vi "WSVCAP SHL FPGA LL Procedure RFFE - Receive Data.vi"(0 "Procedure Step":T1, 1 "Wait Ticks Remaining":u32, 2 "Start of Procedure":bool, 5 "RFFE Wait Ticks":u32, 7 "Read Bits Remaining":u8, 9 "Read Bytes Remaining":u8, 11 "error in (no error)":errorcluster, 12 "RFFE Cycle CMD":u64, 13 "Socket Mask":u64) -> (3 "Wait Ticks Remaining Out":u32, 4 "Procedure Step Out":T1, 6 "Read Bytes Remaining Out":u8, 8 "Read Bits Remaining Out":u8, 10 "Finished":bool, 15 "error out":errorcluster)   [LabVIEW 2017]
uses:
  Type Defs/WSVCAP SHL Procedure Step Enum.ctl
  Type Defs/WSVCAP SHL RFFE Write Line Enum.ctl
  Type Defs/WSVCAP SHL FIFO Operation Enum.ctl
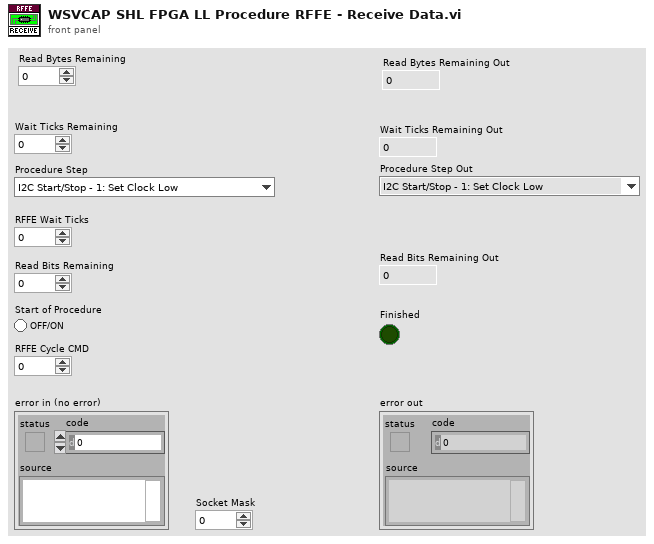
[diagram p1: front panel]
types:
  T1 = typedef "WSVCAP SHL Procedure Step Enum.ctl" = enum16{"I2C Start/Stop - 1: Set Clock Low", "I2C Start/Stop - 2: Wait", "I2C Start/Stop - 3: Set Data I", "I2C Start/Stop - 4: Wait", "I2C Start/Stop - 5: Set Clock High", "I2C Start/Stop - 6: Wait", "I2C Start/Stop - 7: Set Data II", "I2C Start/Stop - 8: Wait", "I2C Start/Stop - 9: Set Clock Low", "I2C Start/Stop - 10: Wait", "I2C Read ACK - 1: Set Clock High", "I2C Read ACK - 2: Wait", "I2C Read ACK - 3: Read ACK Bit", "I2C Read ACK - 4: Wait", "I2C Read ACK - 5: Set Clock Low", "I2C Read ACK - 6: Wait", "I2C Write ACK - 1: Write ACK Bit", "I2C Write ACK - 2: Wait", "I2C Write ACK - 3: Set Clock High", "I2C Write ACK - 4: Wait", "I2C Write ACK - 5: Set Clock Low", "I2C Write ACK - 6: Wait", "I2C Write ACK - 7: Set Data Low", "I2C Send Add - 1: Reset Bits Remaining", "I2C Send Add - 2: Set Data Bit", "I2C Send Add - 3: Wait", "I2C Send Add - 4: Set Clock High", "I2C Send Add - 5: Wait", "I2C Send Add - 6: Set Clock Low", "I2C Send Add - 7: Wait", "I2C Send Add - 8: Check Bits Remaining", "I2C Send Data - 1: Reset Bits Remaining", "I2C Send Data - 2: Load Write Bit from FIFO", "I2C Send Data - 3: Set Data Bit", "I2C Send Data - 4: Wait", "I2C Send Data - 5: Set Clock High", "I2C Send Data - 6: Wait", "I2C Send Data - 7: Set Clock Low", "I2C Send Data - 8: Wait", "I2C Send Data - 9: Check Bits Remaining", "I2C Receive Data - 1: Reset Bits Remaining", "I2C Receive Data - 2: Wait", "I2C Receive Data - 3: Set Clock High", "I2C Receive Data - 4: Wait", "I2C Receive Data - 5: Read Data Bit", "I2C Receive Data - 6: Wait", "I2C Receive Data - 7: Set Clock Low", "I2C Receive Data - 8: Wait", "I2C Receive Data - 9: Check Bits Remaining", "RFFE Send SSC - 1:Set Low", "RFFE Send SSC - 2:Wait", "RFFE Send SSC - 3:Set SDA High", "RFFE Send SSC - 4:Wait", "RFFE Send SSC - 5:Set SDA Low", "RFFE Send SSC - 6:Wait", "RFFE Send Data - 1:Set SCL High", "RFFE Send Data - 2:Wait", "RFFE Send Data - 3:Set SCL Low", "RFFE Send Data - 4:Wait", "RFFE Send Data - 5:Set SCL High (P)", "RFFE Send Data - 6:Wait", "RFFE Send Data - 7:Set SCL Low (P)", "RFFE Send Data - 8:Wait", "RFFE Send Data - 9:Set SCL High (BP)", "RFFE Send Data - 10:Wait", "RFFE Send Data - 11:Set SCL Low (BP)", "RFFE Send Data - 12:Wait", "RFFE Receive Data - 1:Set SCL High", "RFFE Receive Data - 2:Wait", "RFFE Receive Data - 3:Set SCL Low", "RFFE Receive Data - 4:Wait", "RFFE Receive Data - 5:Set SCL High (BP)", "RFFE Receive Data - 6:Wait", "RFFE Receive Data - 7:Set SCL Low (BP)", "RFFE Receive Data - 8:Wait", "RFFE Wait CMD Delay - 1:Wait", "RFFE Clear Lines - 1:Clear"}
  T2 = typedef "WSVCAP SHL RFFE Write Line Enum.ctl" = enum16{"SDAA", "SCLK"}
  T3 = typedef "WSVCAP SHL FIFO Operation Enum.ctl" = enum16{"Create FIFO/Memory", "Get Write FIFO Status", "Get Read FIFO Status", "Put Element in Write", "Put Element in Read", "Get Element from Write", "Get Element from Read"}
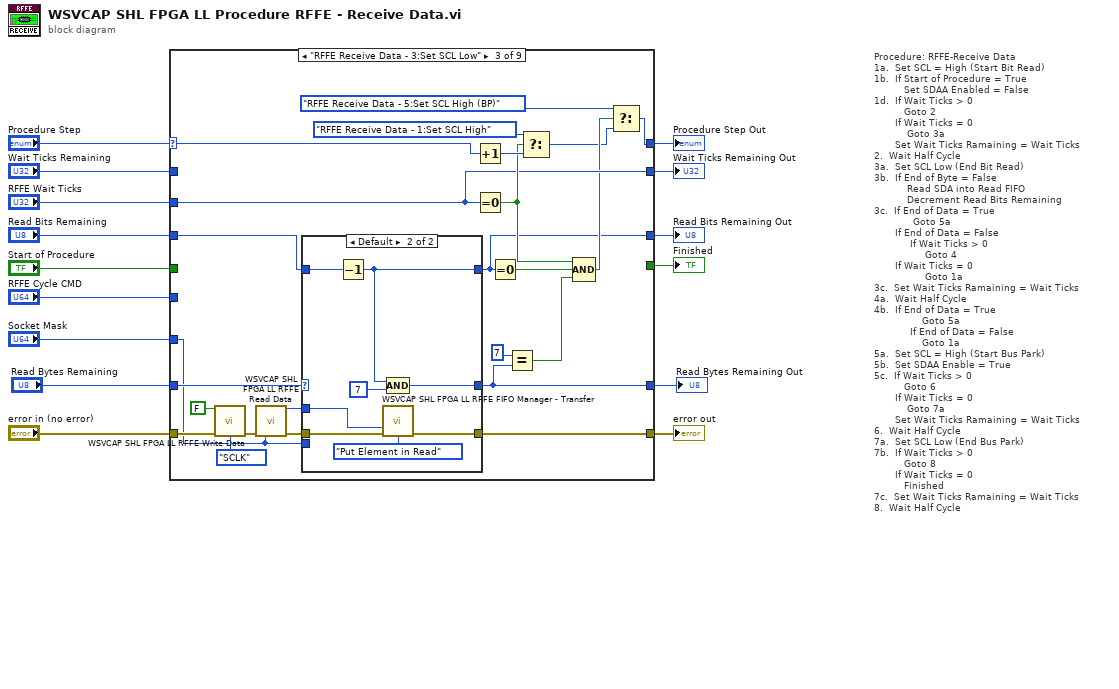
[diagram p0: block diagram]
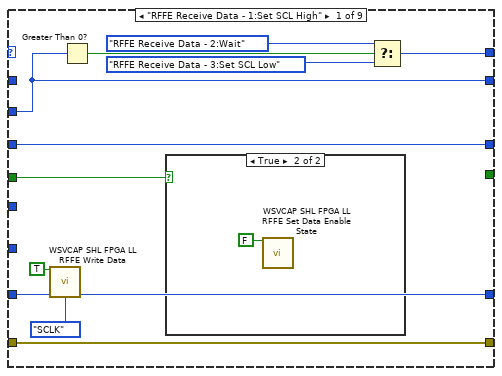
[diagram p2: hidden frame]
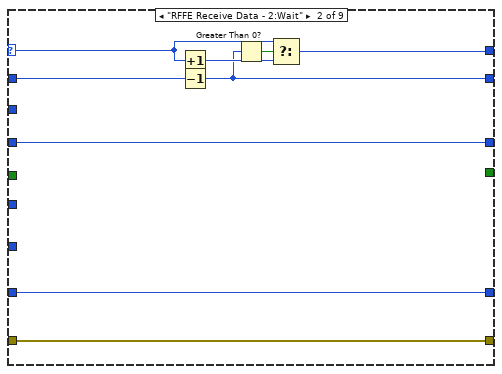
[diagram p4: hidden frame]
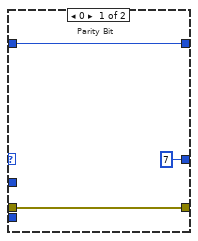
[diagram p5: hidden frame]
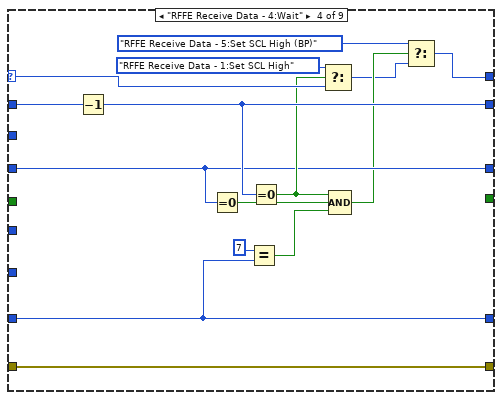
[diagram p6: hidden frame]
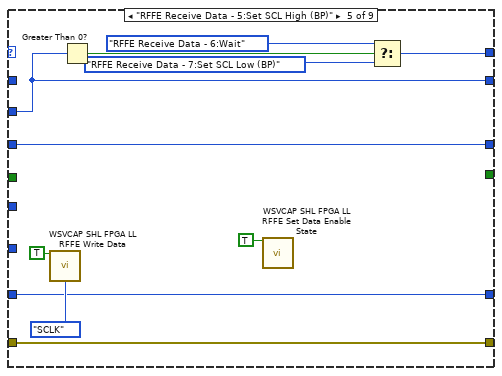
[diagram p7: hidden frame]
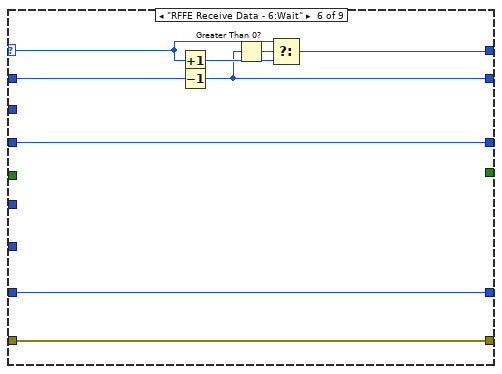
[diagram p8: hidden frame]
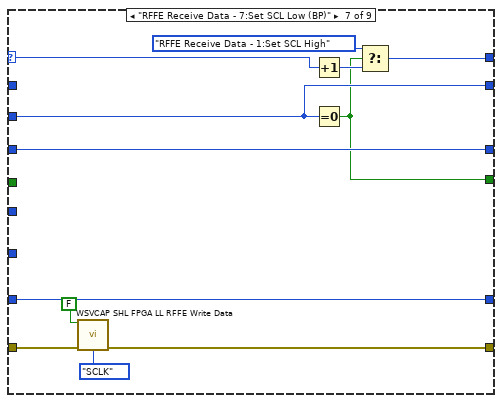
[diagram p9: hidden frame]
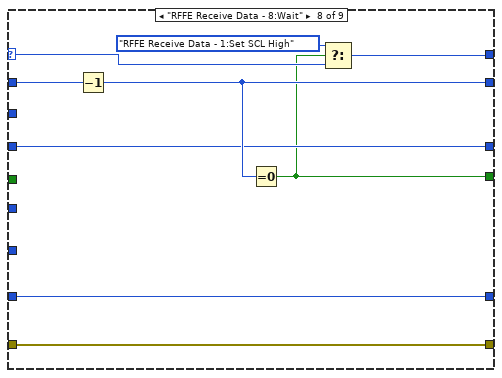
[diagram p10: hidden frame]
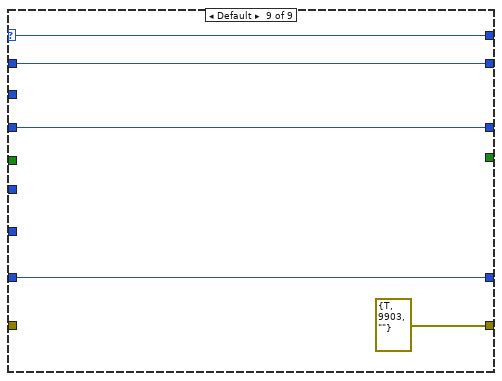
[diagram p11: hidden frame]
diagram:
  # "Procedure: RFFE-Receive Data\n1a.  Set SCL = High (Start Bit Read)\n1b.  If Start of Procedure = True\n          Set SDAA Enabled = False\n1d.  If Wait Ticks > 0\n          Goto 2\n       If Wait Ticks = 0 \n           Goto 3a\n       Set Wait Ticks Ramaining = Wait Ticks\n2.  Wait Half Cycle\n3a.  Set SCL Low (End Bit Read)\n3b.  If End of Byte = False\n           Read SDA into Read FIFO\n           Decrement Read Bits Remaining\n3c.  If End of Data = True\n             Goto 5a\n       If End of Data = False\n            If Wait Ticks > 0\n                 Goto 4\n       If Wait Ticks = 0         \n                 Goto 1a\n3c.  Set Wait Ticks Ramaining = Wait Ticks     \n4a.  Wait Half Cycle\n4b.  If End of Data = True\n                Goto 5a\n            If End of Data = False\n                Goto 1a\n5a.  Set SCL = High (Start Bus Park)\n5b.  Set SDAA Enable = True\n5c.  If Wait Ticks > 0\n          Goto 6\n       If Wait Ticks = 0 \n           Goto 7a\n       Set Wait Ticks Ramaining = Wait Ticks\n6.  Wait Half Cycle\n7a.  Set SCL Low (End Bus Park)\n7b.  If Wait Ticks > 0\n          Goto 8\n       If Wait Ticks = 0 \n          Finished\n7c.  Set Wait Ticks Ramaining = Wait Ticks\n8.  Wait Half Cycle"
  n1 = case shown="\"RFFE Receive Data - 3:Set SCL Low\"" "Procedure Step" {
    selector: "Procedure Step" -> [_ w34 w60 w85 _ w104 w118 w126 w131]
    tunnel: [w23 w36 w55 w86 w94 w106 w110 w127 errorcluster {"status"=TRUE, "code"=9903, "source"=""} ("error IO")] -> w14
    tunnel: "error in (no error)" -> [w23 w36 w56 w86 w94 w106 w114 w127 _]
    tunnel: "Wait Ticks Remaining" -> [_ w32 _ w84 _ w102 _ w125 w130]
    tunnel: "RFFE Wait Ticks" -> [w19 _ w51 _ w90 _ w111 _ _]
    tunnel: [_ _ _ _ _ _ w108 w120 _] -> w13
    tunnel: "Read Bits Remaining" -> [w17 w29 w46 w79 w88 w99 w109 w121 w129]
    tunnel: "Socket Mask" -> [_ _ w37 _ _ _ _ _ _]
    tunnel: "RFFE Cycle CMD" -> [_ _ _ _ _ _ _ _ _]
    tunnel: [w20 w31 w47 w75 w91 w101 w112 w123 w131] -> w7
    tunnel: [w19 w30 w51 w81 w90 w100 w111 w122 w130] -> w6
    tunnel: [w17 w29 w44 w79 w88 w99 w109 w121 w129] -> w5
    tunnel: "Start of Procedure" -> [w18 _ _ _ _ _ _ _ _]
    tunnel: "Read Bytes Remaining" -> [w16 w28 w45 w73 w87 w98 w107 w119 w128]
    tunnel: [w16 w28 w43 w73 w87 w98 w107 w119 w128] -> w2
    frame "RFFE Receive Data - 1:Set SCL High" {
      n2 = call "WSVCAP SHL FPGA LL RFFE Write Data.vi"("Bit In"=TRUE, "Line"=WSVCAP_SHL_RFFE_Write_Line_Enum."SCLK") -> ()  [unwired: 13 in, 1 out]
      n3 = Greater Than 0?(x=w19) -> (x > 0?=w24:bool)
      n4 = case shown="True" w18 {
        frame False {
        }
        frame True {
          n5 = call "WSVCAP SHL FPGA LL RFFE Set Data Enable State.vi"("State"=FALSE) -> ()  [unwired: 14 in, 1 out]
        }
      }
      n6 = Select(t=WSVCAP_SHL_Procedure_Step_Enum."RFFE Receive Data - 2:Wait" ("Procedure Step"), s=w24, f=WSVCAP_SHL_Procedure_Step_Enum."RFFE Receive Data - 3:Set SCL Low" ("Procedure Step")) -> (s? t:f=w20:T1)
    }
    frame "RFFE Receive Data - 2:Wait" {
      n7 = Increment(x=w34) -> (x+1=w33:T1)
      n8 = Decrement(x=w32) -> (x-1=w30:u32)
      n9 = Greater Than 0?(x=w30) -> (x > 0?=w35:bool)
      n10 = Select(t=w34, s=w35, f=w33) -> (s? t:f=w31:T1)
    }
    frame "RFFE Receive Data - 3:Set SCL Low" {
      n11 = call "WSVCAP SHL FPGA LL RFFE Write Data.vi"("Bit In"=FALSE, "error in (no error)"=w56, "Line"=WSVCAP_SHL_RFFE_Write_Line_Enum."SCLK") -> ("error out"=w40:errorcluster)  [unwired: 12 in]
      n12 = call "WSVCAP SHL FPGA LL RFFE Read Data.vi"("error in (no error)"=w40, "Socket Mask"=w37) -> ("Word Out (1-Bit for Each Channel)"=w38:u64, "error out"=w39:errorcluster)  [unwired: 12 in]
      n13 = case shown="Default" w45 {
        tunnel: w39 -> [w63 w65]
        tunnel: [w63 w71] -> w55
        tunnel: w37 -> [_ _]
        tunnel: w46 -> [w62 w69]
        tunnel: [w62 w67] -> w44
        tunnel: [u8 7 w66] -> w43
        tunnel: w38 -> [_ w64]
        frame 0 {
          # "Parity Bit"
        }
        frame Default {
          n14 = Decrement(x=w69) -> (x-1=w67:u8)
          n15 = call "WSVCAP SHL FPGA LL RFFE FIFO Manager - Transfer.vi"("Word In"=w64, "error in (no error)"=w65, "Operation"=WSVCAP_SHL_FIFO_Operation_Enum."Put Element in Read") -> ("error out"=w71:errorcluster)  [unwired: 10 in, 2 out]
          n16 = Compound Arithmetic op=AND(w67, u8 7 ("y")) -> (w66:u8)
        }
      }
      n17 = Increment(x=w60) -> (x+1=w59:T1)
      n18 = Equal To 0?(x=w51) -> (x = 0?=w53:bool)
      n19 = Equal To 0?(x=w44) -> (x = 0?=w54:bool)
      n20 = Equal?(x=u8 7, y=w43) -> (x = y?=w41:bool)
      n21 = Select(t=WSVCAP_SHL_Procedure_Step_Enum."RFFE Receive Data - 1:Set SCL High" ("Procedure Step"), s=w53, f=w59) -> (s? t:f=w48:T1)
      n22 = Compound Arithmetic op=AND(w53, w54, w41) -> (w50:bool)
      n23 = Select(t=WSVCAP_SHL_Procedure_Step_Enum."RFFE Receive Data - 5:Set SCL High (BP)" ("Procedure Step"), s=w50, f=w48) -> (s? t:f=w47:T1)
    }
    frame "RFFE Receive Data - 4:Wait" {
      n24 = Decrement(x=w84) -> (x-1=w81:u32)
      n25 = Equal To 0?(x=w79) -> (x = 0?=w83:bool)
      n26 = Equal?(x=u8 7, y=w73) -> (x = y?=w72:bool)
      n27 = Equal To 0?(x=w81) -> (x = 0?=w80:bool)
      n28 = Select(t=WSVCAP_SHL_Procedure_Step_Enum."RFFE Receive Data - 1:Set SCL High" ("Procedure Step"), s=w80, f=w85) -> (s? t:f=w76:T1)
      n29 = Compound Arithmetic op=AND(w80, w83, w72) -> (w78:bool)
      n30 = Select(t=WSVCAP_SHL_Procedure_Step_Enum."RFFE Receive Data - 5:Set SCL High (BP)" ("Procedure Step"), s=w78, f=w76) -> (s? t:f=w75:T1)
    }
    frame "RFFE Receive Data - 5:Set SCL High (BP)" {
      n31 = call "WSVCAP SHL FPGA LL RFFE Write Data.vi"("Bit In"=TRUE, "Line"=WSVCAP_SHL_RFFE_Write_Line_Enum."SCLK") -> ()  [unwired: 13 in, 1 out]
      n32 = Greater Than 0?(x=w90) -> (x > 0?=w95:bool)
      n33 = call "WSVCAP SHL FPGA LL RFFE Set Data Enable State.vi"("State"=TRUE) -> ()  [unwired: 14 in, 1 out]
      n34 = Select(t=WSVCAP_SHL_Procedure_Step_Enum."RFFE Receive Data - 6:Wait" ("Procedure Step"), s=w95, f=WSVCAP_SHL_Procedure_Step_Enum."RFFE Receive Data - 7:Set SCL Low (BP)" ("Procedure Step")) -> (s? t:f=w91:T1)
    }
    frame "RFFE Receive Data - 6:Wait" {
      n35 = Increment(x=w104) -> (x+1=w103:T1)
      n36 = Decrement(x=w102) -> (x-1=w100:u32)
      n37 = Greater Than 0?(x=w100) -> (x > 0?=w105:bool)
      n38 = Select(t=w104, s=w105, f=w103) -> (s? t:f=w101:T1)
    }
    frame "RFFE Receive Data - 7:Set SCL Low (BP)" {
      n39 = call "WSVCAP SHL FPGA LL RFFE Write Data.vi"("Bit In"=FALSE, "error in (no error)"=w114, "Line"=WSVCAP_SHL_RFFE_Write_Line_Enum."SCLK") -> ("error out"=w110:errorcluster)  [unwired: 12 in]
      n40 = Increment(x=w118) -> (x+1=w117:T1)
      n41 = Equal To 0?(x=w111) -> (x = 0?=w108:bool)
      n42 = Select(t=WSVCAP_SHL_Procedure_Step_Enum."RFFE Receive Data - 1:Set SCL High" ("Procedure Step"), s=w108, f=w117) -> (s? t:f=w112:T1)
    }
    frame "RFFE Receive Data - 8:Wait" {
      n43 = Decrement(x=w125) -> (x-1=w122:u32)
      n44 = Equal To 0?(x=w122) -> (x = 0?=w120:bool)
      n45 = Select(t=WSVCAP_SHL_Procedure_Step_Enum."RFFE Receive Data - 1:Set SCL High" ("Procedure Step"), s=w120, f=w126) -> (s? t:f=w123:T1)
    }
    frame Default {
    }
  }
  "error out" <- w14
  "Finished" <- w13
  "Procedure Step Out" <- w7
  "Wait Ticks Remaining Out" <- w6
  "Read Bits Remaining Out" <- w5
  "Read Bytes Remaining Out" <- w2
